vi "Create_NMR_waveform.vi"(10 "time":timestamp, 11 "Y data":dbl) -> (3 "waveform_array":waveform(dbl)[](array[waveform])=[{"t0"=timestamp(0 s since 1904-01-01), "dt"=1.0, "Y"=[]}, {"t0"=timestamp(3732035173.078092 s since 1904-01-01), "dt"=1.0, "Y"=[302.8589782714844], "attributes"=variant("NI_ChannelName"=variant(string "T1"))}])   [LabVIEW 2019]
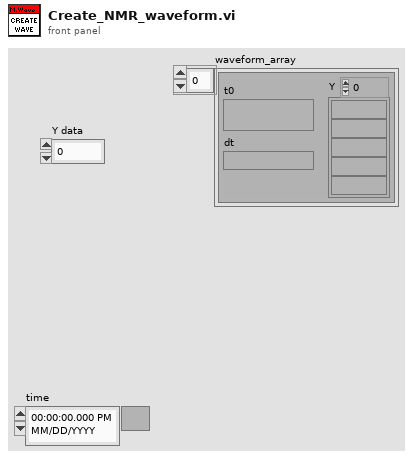
[diagram p1: front panel]
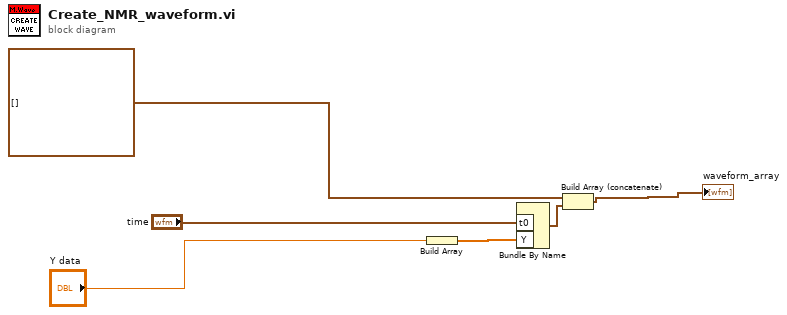
[diagram p0: block diagram]
diagram:
  n1 = Build Array("Y data") -> (w2:dbl[])
  n2 = Bundle By Name("t0"="time", "Y"=w2) -> (w3:waveform(dbl))  [unwired: 1 in]
  n3 = Build Array (concatenate)(waveform(dbl)[] [], w3) -> (→"waveform_array":waveform(dbl)[])
